vi "数组元素标签.vi"() -> ()   [LabVIEW 2012]
panel:
  out "Daq":cluster{"字符串 2":string, "数值":dbl}[](array[cluster])
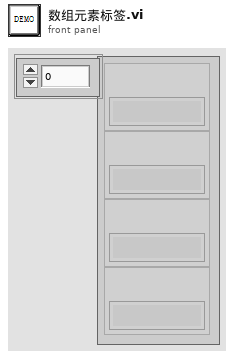
[diagram p1: front panel]
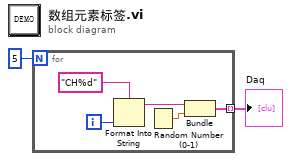
[diagram p0: block diagram]
diagram:
  n1 = for {
    N: 5 -> [_]
    tunnel: [w3] -> w1 mode=indexing
    i -> [w7]
    n2 = Format Into String(format string="CH%d" ("格式字符串"), w7) -> (resulting string=w5:string)  [unwired: 2 in, 1 out]
    n3 = Random Number (0-1)() -> (number: 0 to 1=w4:dbl)
    n4 = Bundle(w5, "number: 0 to 1"=w4) -> (w3:cluster{string, "number: 0 to 1":dbl})  [unwired: 1 in]
  }
  "Daq" <- w1
